vi "PlLoN_grabber2.vi"(7 "Number of Images":u32=1 min=1 step=1, 8 "error in (no error)":errorcluster, 11 "Camera Handle":u32) -> (0 "error out":errorcluster, 1 "DATA":u16[][](array[numeric]), 2 "Number of Images":u32=1 min=1 step=1, 3 "Camera Handle":u32, 4 "x/y":dbl)   [LabVIEW 2014]
panel:
  out "Waveform Graph":u16[](graph)
  out "PyLoN Ready":bool
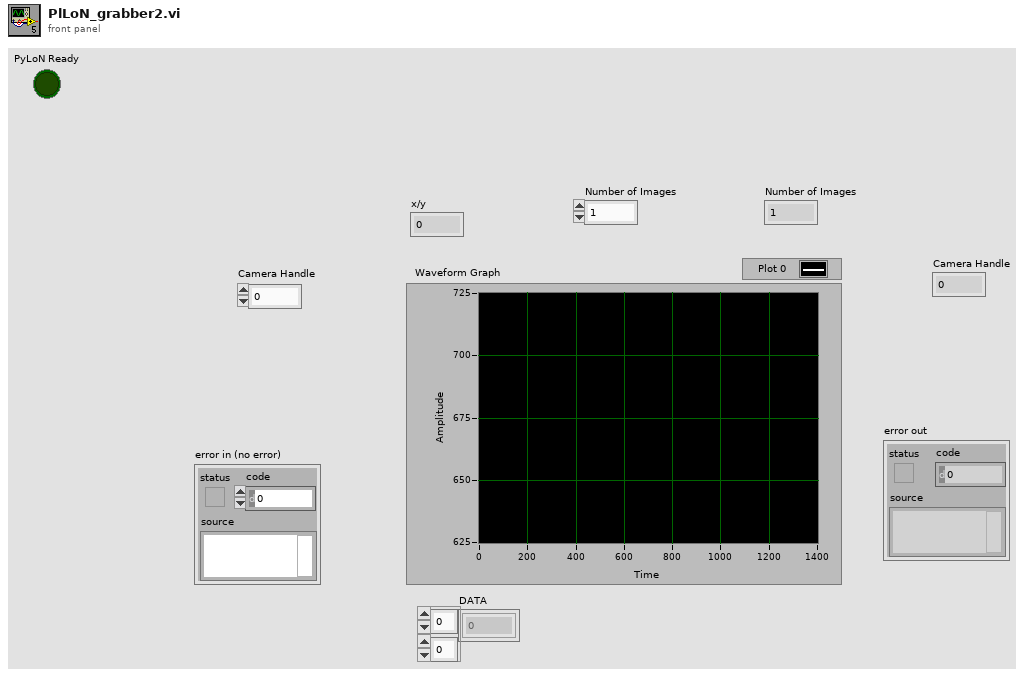
[diagram p1: front panel]
types:
  T1 = cluster{"Camera Handle":u32, "Pulser Handle":u32, "File Handle":u32, "Display Handle":u32, "Image Handle":u32}
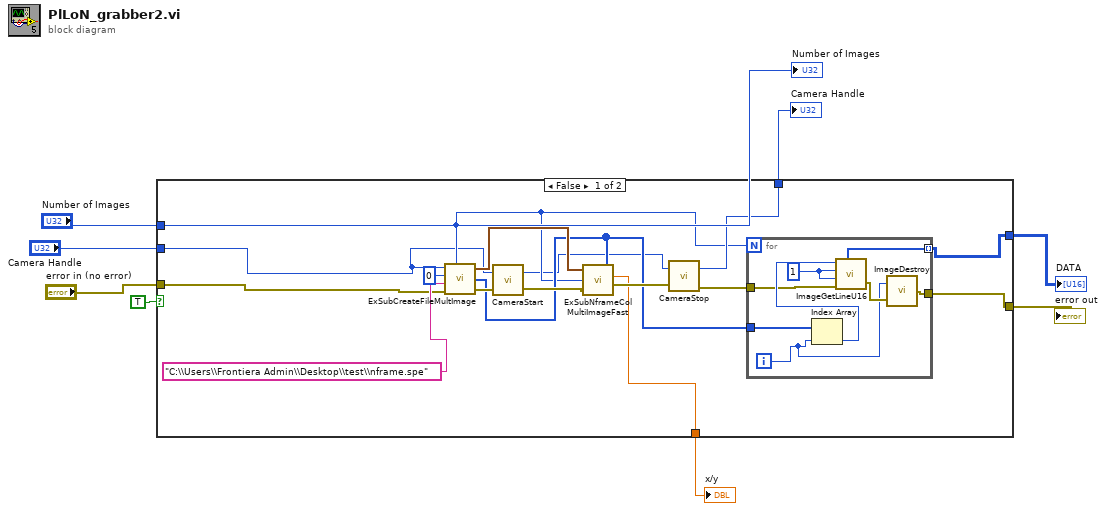
[diagram p0: block diagram]
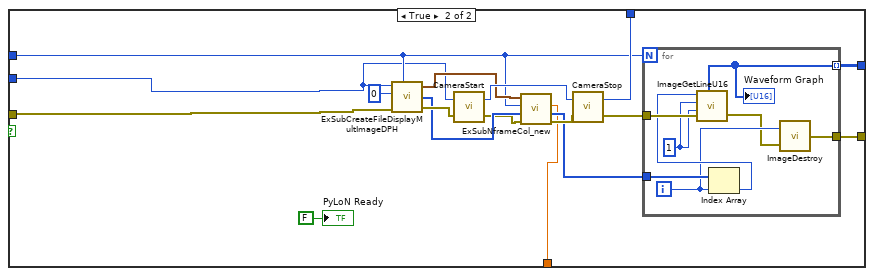
[diagram p2: hidden frame]
diagram:
  n1 = case shown="False" TRUE {
    tunnel: [w16 w46] -> w8
    tunnel: [w14 w45] -> w7
    tunnel: [w15 w42] -> w6
    tunnel: "Number of Images" -> [w12 w40]
    tunnel: [w13 w35] -> w5
    tunnel: "error in (no error)" -> [w10 w34]
    tunnel: "Camera Handle" -> [w9 w33]
    frame False {
      n2 = call "ExSubCreateFileMultImage.vi"("Camera Handle"=w9, "Pulser Handle"=u32 0, "File and Display Name"="C:\\Users\\Frontiera Admin\\Desktop\\test\\nframe.spe", "error in (no error)"=w10, "Number of Images"=w12) -> ("Handles Out"=w20:T1, "Array"=w18:u32[], "error out"=w22:errorcluster)
      n3 = call <userlib>:"CameraStart.vi"("error in"=w22, "Camera Handle"=w9) -> ("error out"=w21:errorcluster, "Camera Handle"=w11:u32)
      n4 = call "ExSubNframeColMultiImageFast.vi"("Handle Cluster"=w20, "Number of Images"=w12, "error in (no error)"=w21, "image handles"=w18) -> ("x/y"=w13:dbl, "error out"=w19:errorcluster)  [unwired: 1 out]
      n5 = call <userlib>:"CameraStop.vi"("error in"=w19, "Camera Handle"=w11) -> ("error out"=w17:errorcluster, "Camera Handle"=w14:u32)
      n6 = for {
        N: w12 -> [_]
        tunnel: w18 -> [w32]
        tunnel: w17 -> [w29]
        tunnel: [w28] -> w16 mode=indexing
        tunnel: [w26] -> w15
        i -> [w25]
        w30 = u32 1 ("Y Position")
        n7 = Index Array(array=w32, index=w25) -> (element=w31:u32)
        n8 = call <userlib>:"ImageGetLineU16.vi"("Data Handle"=w31, "Y Position"=w30, "Z Position"=w30, "error in"=w29) -> ("Array u16"=w28:u16[], "error out"=w27:errorcluster)  [unwired: 1 out]
        n9 = call <userlib>:"ImageDestroy.vi"("error in"=w27, "Data handle"=w25) -> ("error out"=w26:errorcluster)
      }
    }
    frame True {
      n10 = call "ExSubCreateFileDisplayMultImageDPH.vi"("Camera Handle"=w33, "Pulser Handle"=u32 0, "error in (no error)"=w34, "Number of Images"=w40) -> ("Handles Out"=w41:T1, "Array"=w39:u32[], "error out"=w44:errorcluster)  [unwired: 1 in]
      n11 = call <userlib>:"CameraStart.vi"("error in"=w44, "Camera Handle"=w33) -> ("error out"=w38:errorcluster, "Camera Handle"=w47:u32)
      n12 = call "ExSubNframeCol_new.vi"("error in (no error)"=w38, "image handles"=w39, "Number of Images"=w40, "Handle Cluster 2"=w41) -> ("error out"=w37:errorcluster, "data handles"=w36:u32[], "x/y"=w35:dbl)  [unwired: 4 in, 1 out]
      n13 = call <userlib>:"CameraStop.vi"("error in"=w37, "Camera Handle"=w47) -> ("error out"=w48:errorcluster, "Camera Handle"=w45:u32)
      n14 = for {
        N: w40 -> [_]
        tunnel: w36 -> [w53]
        tunnel: w48 -> [w57]
        tunnel: [w54] -> w46 mode=indexing
        tunnel: [w50] -> w42
        i -> [w52]
        w56 = u32 1
        n15 = Index Array(array=w53, index=w52) -> (element=w55:u32)
        n16 = call <userlib>:"ImageGetLineU16.vi"("Data Handle"=w55, "Y Position"=w56, "Z Position"=w56, "error in"=w57) -> ("Array u16"=w54:u16[], "error out"=w51:errorcluster)  [unwired: 1 out]
        "Waveform Graph" <- w54
        n17 = call <userlib>:"ImageDestroy.vi"("error in"=w51, "Data handle"=w52) -> ("error out"=w50:errorcluster)
      }
      "PyLoN Ready" <- FALSE ("PyLoN Ready")
    }
  }
  "error out" <- w6
  "DATA" <- w8
  "Camera Handle" <- w7
  "x/y" <- w5
  "Number of Images" <- "Number of Images"
